vi "WriteToRandomFile.vi"() -> ()   [LabVIEW 2026]
panel:
  out "true":bool
  in  "message":string
  in  "button name (\"OK\")":string
  out "text":string
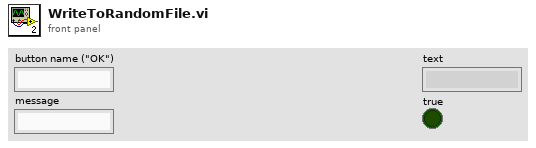
[diagram p1: front panel]
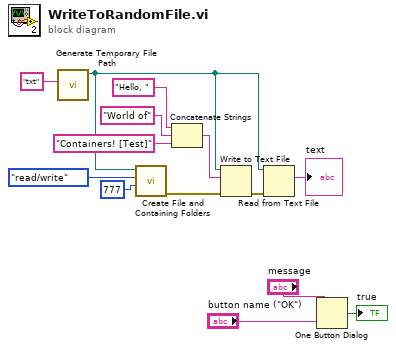
[diagram p0: block diagram]
diagram:
  n1 = call <vilib>:"Generate Temporary File Path.vi"("Temporary File Extension (tmp)"="txt") -> ("Unique Temporary File Path"=w4:path)  [unwired: 9 in, 1 out]
  n2 = call <vilib>:"Create File and Containing Folders.vi"("permissions"=i16 777, "access"=enum16{"read/write", "read-only", "write-only"}."read/write", "file path"=w4) -> ("error out"=w8:errorcluster)  [unwired: 7 in, 1 out]
  n3 = Concatenate Strings("Hello, " ("string"), "World of" ("string"), "Containers! [Test]" ("string")) -> (w7:string)
  n4 = Write to Text File(file (use dialog)=w4, text=w7, error in=w8) -> (error out=w5:errorcluster)  [unwired: 1 in, 2 out]
  n5 = Read from Text File(file (use dialog)=w4, error in=w5) -> (text=→"text":string)  [unwired: 2 in, 3 out]
  n6 = One Button Dialog(message="message", button name ("OK")="button name (\"OK\")") -> (true=→"true":bool)
